vi "Software Update HCC Get Paths.vi"(8 "Error In":errorcluster, 11 "Newfi Exe Folder Path":path=path "C:/Newfi Exe") -> (0 "Error Out":errorcluster, 2 "Stations and Board IDs":path, 3 "Newfi Exe Locations":path)   [LabVIEW 2016]
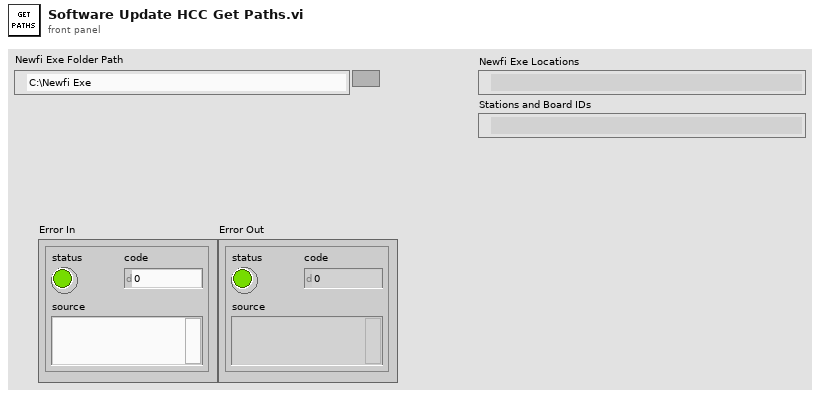
[diagram p1: front panel]
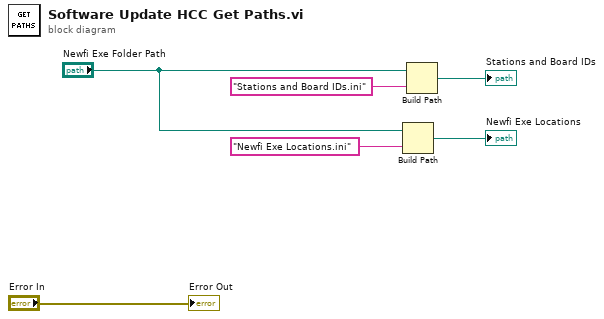
[diagram p0: block diagram]
diagram:
  n1 = Build Path(base path="Newfi Exe Folder Path", name or relative path="Newfi Exe Locations.ini") -> (appended path=→"Newfi Exe Locations":path)
  n2 = Build Path(base path="Newfi Exe Folder Path", name or relative path="Stations and Board IDs.ini") -> (appended path=→"Stations and Board IDs":path)
  "Error Out" <- "Error In"
